vi "Image Analysis.vi"(0 "Color Mode (Color Threshold 1)":u16(ring) items=["RGB", "HSL", "HSV", "HSI"], 4 "Image In":T1(plugin-control), 5 "Blue or Luma or Val or Inten Range":cluster{"Lower value":i32, "Upper value":i32}={"Lower value"=200, "Upper value"=240}, 6 "Green or Sat Range":cluster{"Lower value":i32, "Upper value":i32}={"Lower value"=200, "Upper value"=255}, 7 "Red or Hue Range":cluster{"Lower value":i32, "Upper value":i32}={"Lower value"=200, "Upper value"=255}) -> (1 "error out":errorcluster, 2 "Y Centroid":sgl, 3 "X Centroid":sgl)   [LabVIEW 2013]
panel:
  out "Image Out":T1(plugin-control)
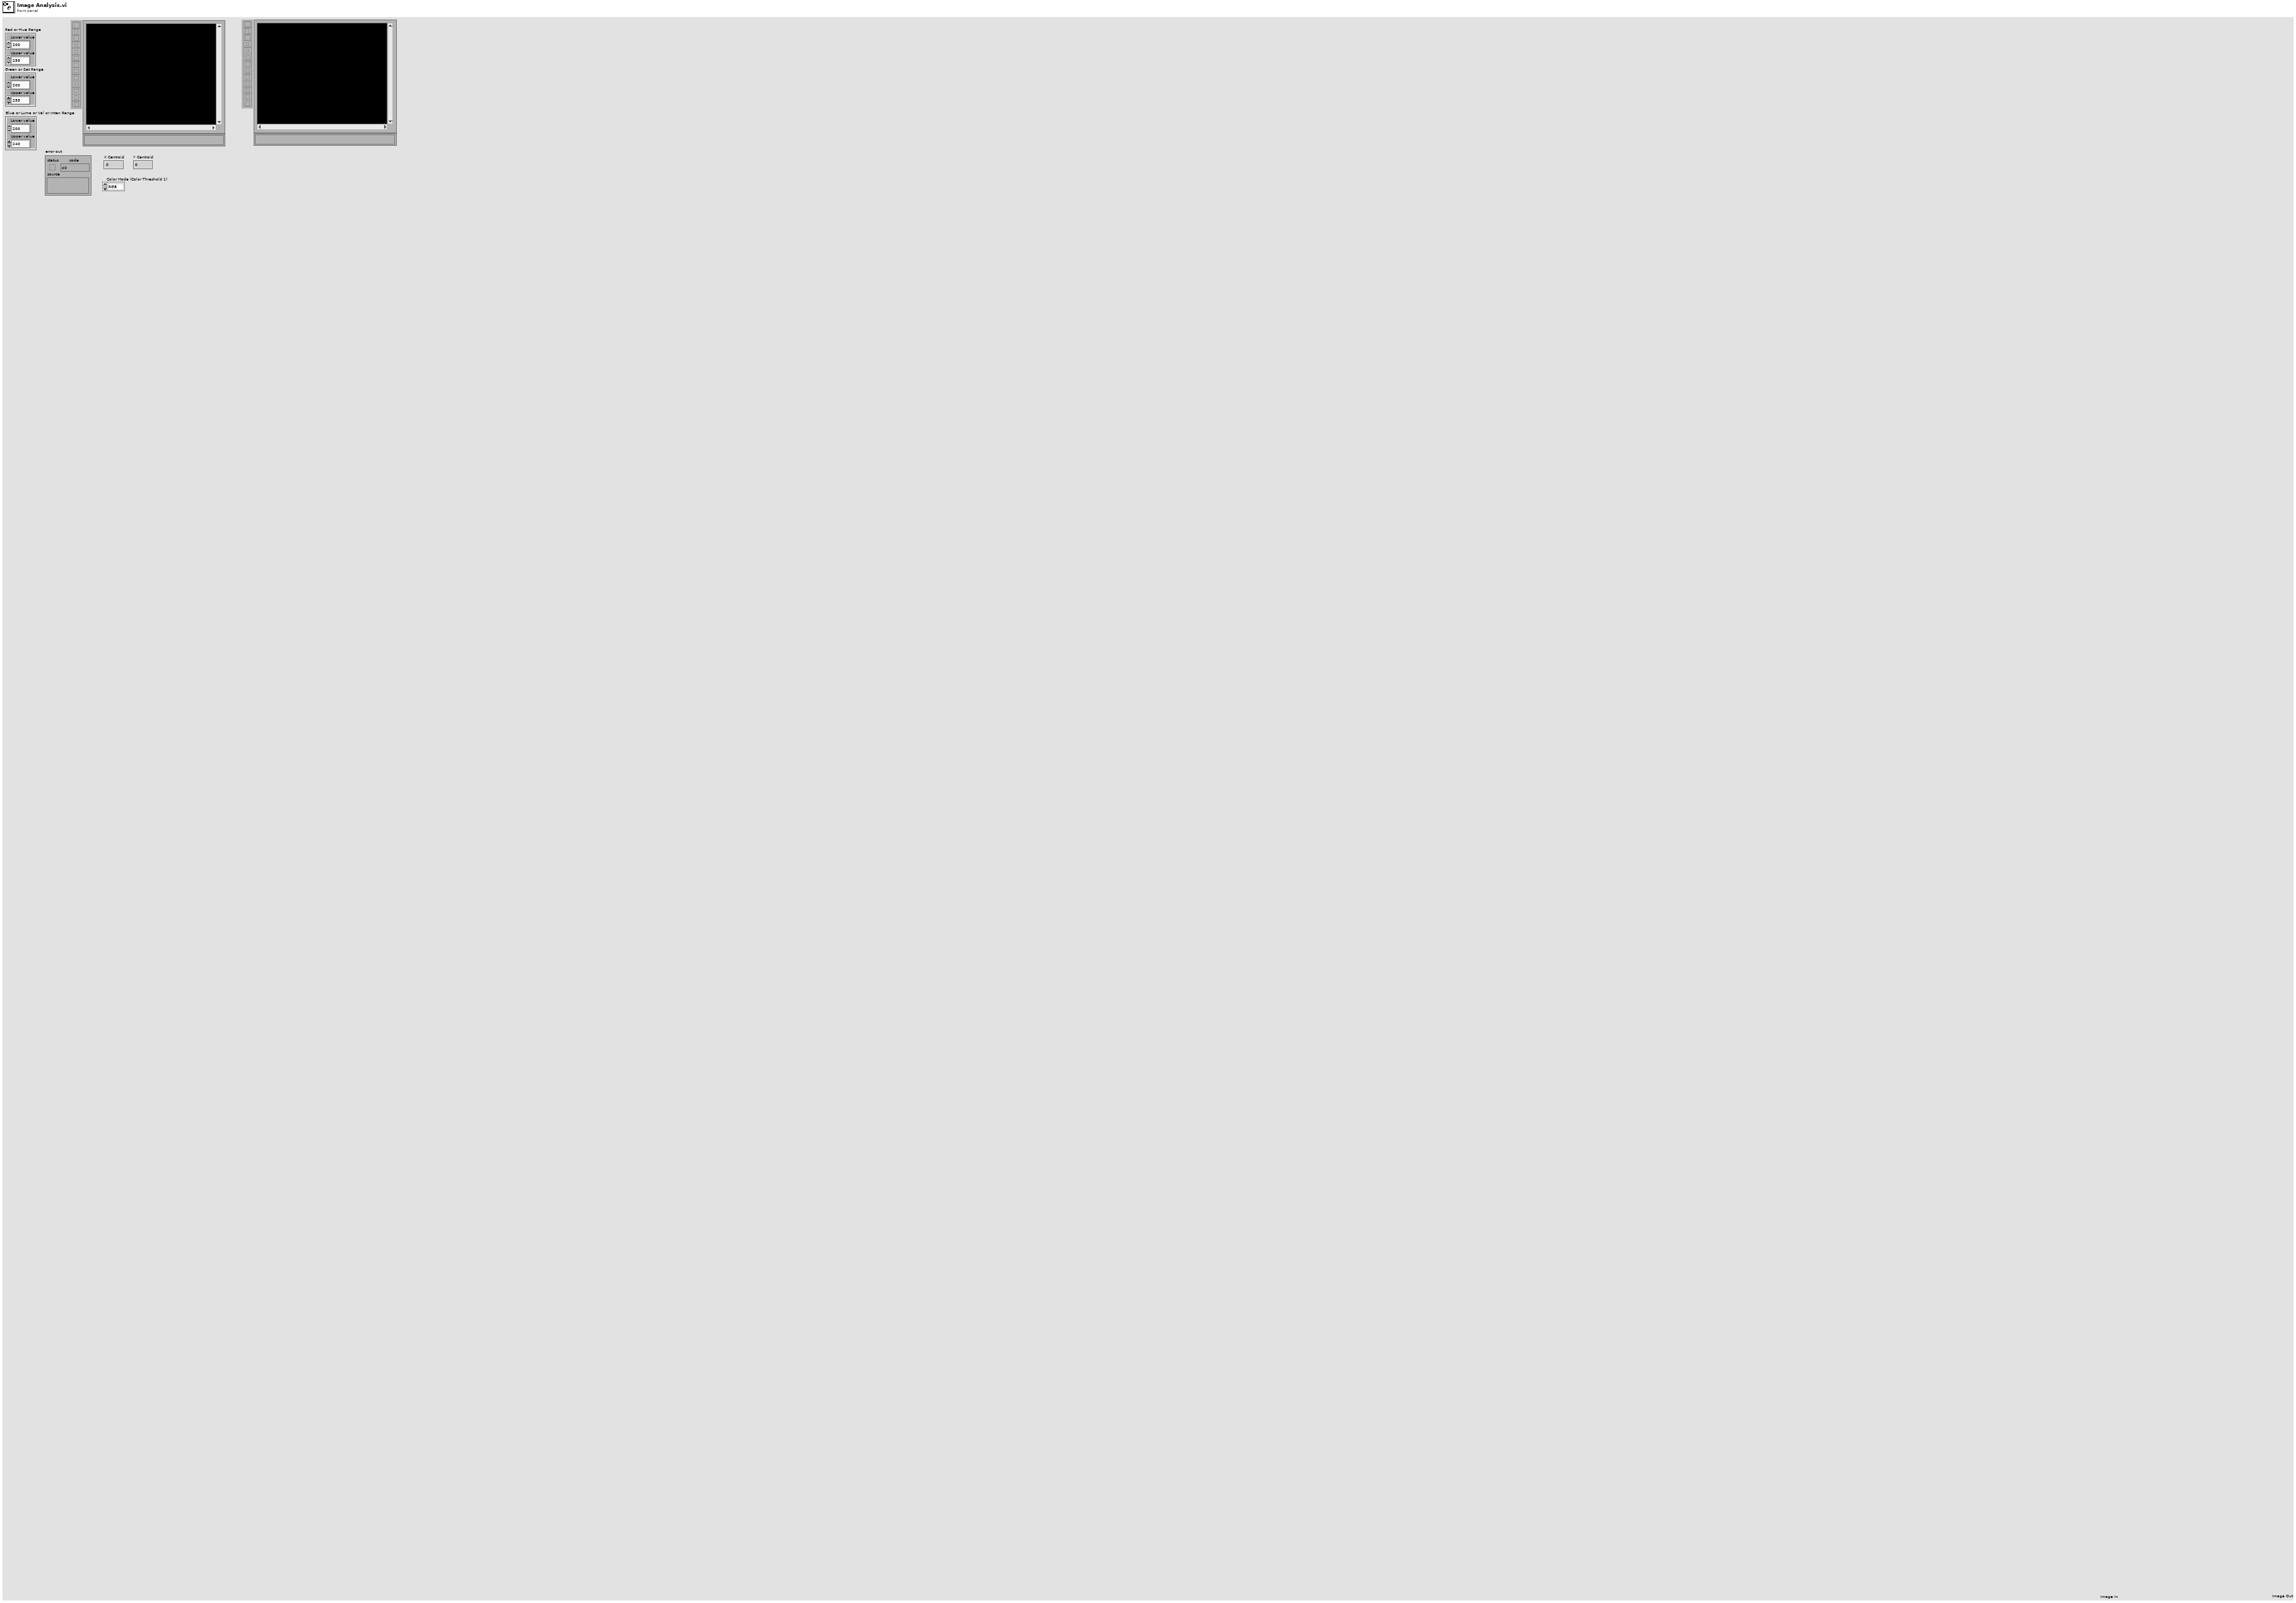
[diagram p1: front panel]
types:
  T1 = typedef "IMAQ Image.ctl" = refnum<image>
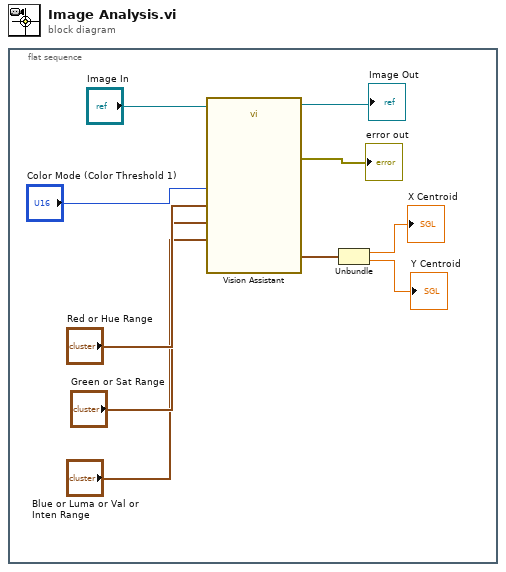
[diagram p0: block diagram]
diagram:
  n1 = flat-sequence {
    frame #0 {
      n2 = call "Vision Assistant"("Image In"="Image In", "Color Mode (Color Threshold 1)"="Color Mode (Color Threshold 1)", "Red or Hue Range (Color Threshold 1)"="Red or Hue Range", "Green or Sat Range (Color Threshold 1)"="Green or Sat Range", "Blue or Luma or Val or Inten Range (Color Threshold 1)"="Blue or Luma or Val or Inten Range") -> ("Image Out"=→"Image Out":T1, "Centroid (Arrow Centroid)"=w9:cluster{"X Centroid":sgl, "Y Centroid":sgl}, "error out"=→"error out":errorcluster)  [unwired: 20 in]
      n3 = Unbundle(w9) -> ("X Centroid"=→"X Centroid":sgl, "Y Centroid"=→"Y Centroid":sgl)
    }
  }
